vi "Create_WF.vi"(8 "error in":errorcluster caption="entrée d'erreur", 11 "Scanning cluster":T1={"Nx"=4, "Ny"=4, "# Repetition"=1, "FOV_X (µm)"=100.0, "FOV_Y (µm)"=100.0, "Calib_X"=0.1, "Calib_Y"=0.1, "Center X (µm)"=50.0, "Center_Y (µm)"=50.0, "Bi-directionnal?"=FALSE} {"# Repetition" min=1 step=1; "Ny" min=1 step=1; "Nx" min=1 step=1}) -> (0 "error out":errorcluster caption="sortie d'erreur", 2 "Graphe":dbl[][](graph), 3 "Scanning positions":dbl[][](array[numeric])=[[0.0, 3.333333333333333, 6.666666666666666, 10.0, 0.0, 3.333333333333333, 6.666666666666666, 10.0, 0.0, 3.333333333333333, 6.666666666666666, 10.0, 0.0, 3.333333333333333, 6.666666666666666, 10.0], [0.0, 0.0, 0.0, 0.0, 3.333333333333333, 3.333333333333333, 3.333333333333333, 3.333333333333333, 6.666666666666666, 6.666666666666666, 6.666666666666666, 6.666666666666666, 10.0, 10.0, 10.0, 10.0]])   [LabVIEW 2026]
panel:
  out "taille(s)":i32[](array[numeric])
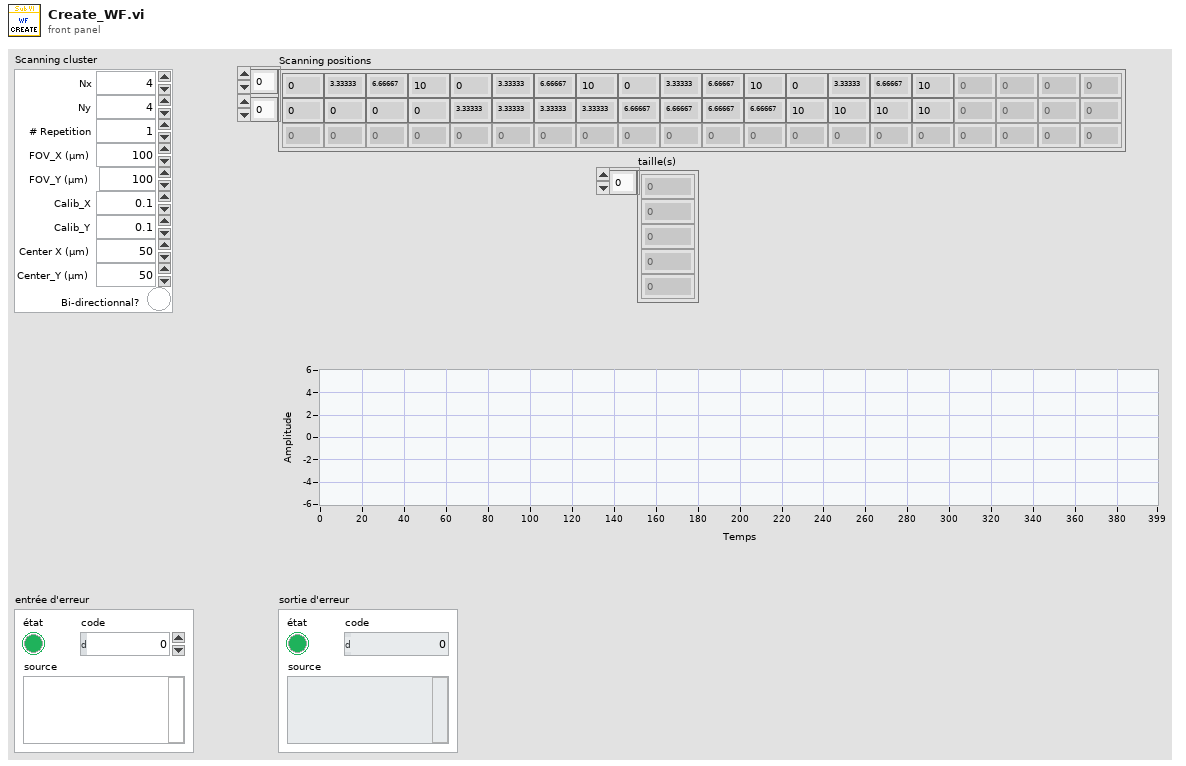
[diagram p1: front panel]
types:
  T1 = cluster{"Nx":u16, "Ny":u16, "# Repetition":u16, "FOV_X (µm)":dbl, "FOV_Y (µm)":dbl, "Calib_X":dbl, "Calib_Y":dbl, "Center X (µm)":dbl, "Center_Y (µm)":dbl, "Bi-directionnal?":bool}
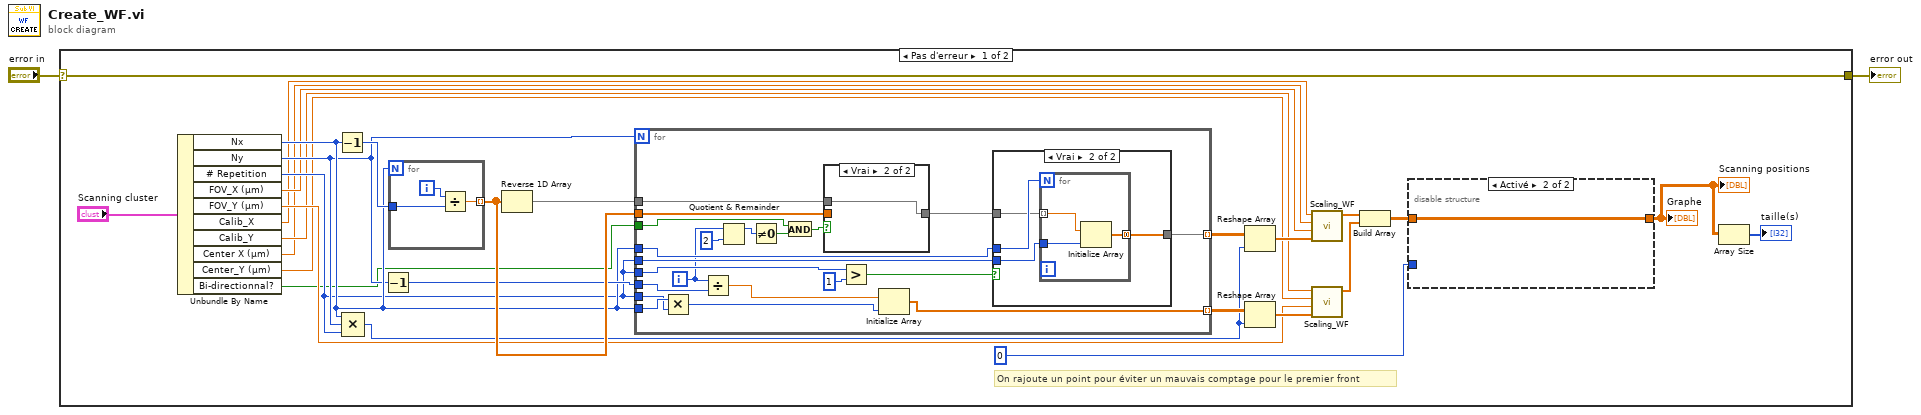
[diagram p0: block diagram]
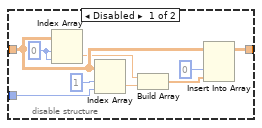
[diagram p2: hidden frame]
diagram:
  n1 = case shown="Pas d'erreur" "error in" {
    selector: "error in" -> [w29 w74]
    tunnel: [w29 w74] -> w1
    frame No Error {
      # "On rajoute un point pour éviter un mauvais comptage pour le premier front"
      n2 = Unbundle By Name("Scanning cluster") -> ("Nx"=w16:u16, "Ny"=w15:u16, "# Repetition"=w14:u16, "FOV_X (µm)"=w13:dbl, "FOV_Y (µm)"=w12:dbl, "Calib_X"=w11:dbl, "Calib_Y"=w10:dbl, "Center X (µm)"=w9:dbl, "Center_Y (µm)"=w8:dbl, "Bi-directionnal?"=w7:bool)
      n3 = Decrement(x=w16) -> (x-1=w28:u16)
      n4 = Compound Arithmetic op=MULTIPLY(w16, w15, w14) -> (w22:u16)
      n5 = Decrement(x=w15) -> (x-1=w25:u16)
      n6 = for {
        N: w16 -> [_]
        tunnel: w28 -> [w72]
        tunnel: [w71] -> w27 mode=indexing
        i -> [w73]
        n7 = Divide(x=w73, y=w72) -> (x/y=w71:dbl)
      }
      n8 = Reverse 1D Array(array=w27) -> (reversed array=w26:dbl[])
      n9 = for {
        N: w15 -> [_]
        tunnel: w7 -> [w58]
        tunnel: w27 -> [w55]
        tunnel: w26 -> [w54]
        tunnel: w14 -> [w53]
        tunnel: w16 -> [w49]
        tunnel: w14 -> [w48]
        tunnel: w25 -> [w47]
        tunnel: w16 -> [w44]
        tunnel: w14 -> [w43]
        tunnel: [w41] -> w24 mode=indexing
        tunnel: [w40] -> w23 mode=indexing
        i -> [w46]
        n10 = Multiply(x=w44, y=w43) -> (x*y=w42:u16)
        n11 = Divide(x=w46, y=w47) -> (x/y=w45:dbl)
        n12 = Quotient & Remainder(x=w46, y=2) -> (x-y*floor(x/y)=w59:i32)  [unwired: 1 out]
        n13 = Not Equal To 0?(x=w59) -> (x != 0?=w60:bool)
        n14 = And(x=w58, y=w60) -> (x .and. y?=w57:bool)
        n15 = case shown="Vrai" w57 {
          tunnel: [w69 w70] -> w50
          tunnel: w55 -> [w69 _]
          tunnel: w54 -> [_ w70]
          frame False {
          }
          frame True {
          }
        }
        n16 = Greater?(x=w53, y=u16 1) -> (0:w51:bool)
        n17 = Initialize Array(w45, w42) -> (w40:dbl[])
        n18 = case shown="Vrai" w51 {
          tunnel: [w61 w62] -> w41
          tunnel: w50 -> [w61 w64]
          tunnel: w49 -> [_ w65]
          tunnel: w48 -> [_ w63]
          frame False {
          }
          frame True {
            n19 = for {
              N: w65 -> [_]
              tunnel: w64 -> [w68] mode=indexing
              tunnel: w63 -> [w67]
              tunnel: [w66] -> w62 mode=concatenating
              n20 = Initialize Array(w68, w67) -> (w66:dbl[])
            }
          }
        }
      }
      n21 = Reshape Array(w24, w22) -> (w21:dbl[])
      n22 = Reshape Array(w23, w22) -> (w19:dbl[])
      n23 = call "Scaling_WF.vi"("Axis_unit_1D"=w21, "FOV_Axis (µm)"=w13, "Center Axis (µm)"=w9, "Calib_Axis"=w11) -> ("Axis_volts"=w20:dbl[])  [unwired: 7 in]
      n24 = call "Scaling_WF.vi"("Axis_unit_1D"=w19, "FOV_Axis (µm)"=w12, "Center Axis (µm)"=w8, "Calib_Axis"=w10) -> ("Axis_volts"=w18:dbl[])  [unwired: 7 in]
      n25 = Build Array(w20, w18) -> (w6:dbl[][])
      n26 = disable-structure shown="Activé" {
        disable-tunnel: w6 -> [w36 w39]
        disable-tunnel: 0 ("indice désactivé (col)") -> [w35 _]
        disable-tunnel: [w30 w39] -> w3
        frame Disabled {
          w38 = 0 ("indice (ligne)")
          n27 = Index Array(array=w36, index (row)=w38, index (col)=w38) -> (element=w34:dbl)
          n28 = Index Array(array=w36, index (row)=1 ("indice (ligne)"), index (col)=w35) -> (element=w33:dbl)
          n29 = Build Array(w34, w33) -> (w32:dbl[])
          n30 = Insert Into Array(array=w36, index (col)=0 ("indice (ligne)"), new element=w32) -> (w30:dbl[][])  [unwired: 1 in]
        }
        frame Enabled {
        }
      }
      "Scanning positions" <- w3
      "Graphe" <- w3
      n31 = Array Size(array=w3) -> (size(s)=→"taille(s)":i32[])
    }
    frame Error {
    }
  }
  "error out" <- w1
